vi "saveLogEntry.vi"(8 "error in (no error)":errorcluster, 11 "TestDataLog in":refnum<class "TestDataLog.lvclass">) -> (0 "error out":errorcluster, 3 "TestDataLog out":refnum<class "TestDataLog.lvclass">)   [LabVIEW 2016, in "TestDataLog.lvclass"]
uses:
  TestDataLog.lvclass
  D:/Code/ts_dcabt/Common_Log/Log/Log.lvclass
  TestDataLog.lvclass/TestDataLog.ctl
  Common_Log/Log/Log.lvclass/Log.ctl
  Common_Log/Log/Log.lvclass
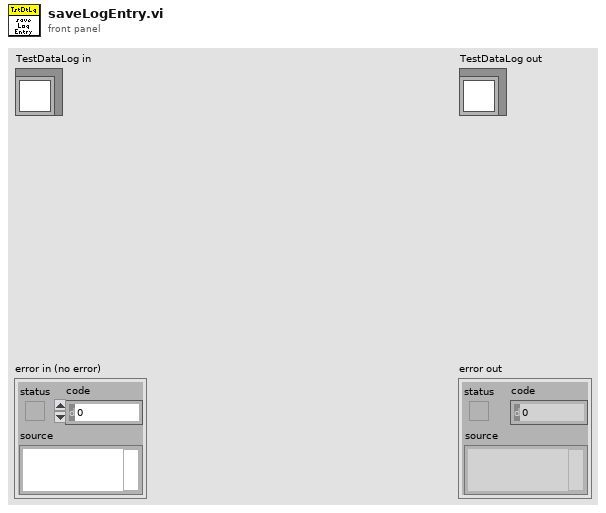
[diagram p1: front panel]
types:
  T1 = typedef "ILCBTTypedefs.lvlib/OutputData.ctl" = cluster{"Ch1":u16, "Ch2":u16, "Ch3":u16}
  T2 = typedef "ILCBTTypedefs.lvlib/StateSelector.ctl" = enum16{"EnabledState", "FaultState", "OffState", "StandbyState", "WaitingForTestState", "ExecutingTestState"}
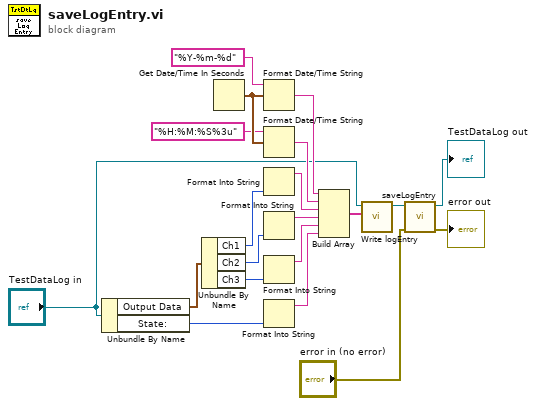
[diagram p0: block diagram]
diagram:
  n1 = Unbundle By Name("TestDataLog in") -> ("Output Data"=w20:T1, "State:"=w17:T2)
  n2 = Unbundle By Name(w20) -> ("Ch1"=w19:u16, "Ch2"=w5:u16, "Ch3"=w2:u16)
  n3 = Get Date/Time In Seconds() -> (seconds since 1Jan1904=w14:timestamp)
  n4 = Format Date/Time String(time format string (%c)="%Y-%m-%d" ("format string"), seconds (now)=w14) -> (date/time string=w11:string)  [unwired: 1 in]
  n5 = Format Date/Time String(time format string (%c)="%H:%M:%S%3u", seconds (now)=w14) -> (date/time string=w12:string)  [unwired: 1 in]
  n6 = Format Into String(w19) -> (resulting string=w18:string)  [unwired: 3 in, 1 out]
  n7 = Format Into String(w5) -> (resulting string=w4:string)  [unwired: 3 in, 1 out]
  n8 = Format Into String(w2) -> (resulting string=w3:string)  [unwired: 3 in, 1 out]
  n9 = Format Into String(w17) -> (resulting string=w16:string)  [unwired: 3 in, 1 out]
  n10 = Build Array(w11, w12, w18, w4, w3, w16) -> (w9:string[])
  n11 = call "Write logEntry.vi"("logEntry"=w9, "Logger in"="TestDataLog in") -> ("Logger out"=w10:refnum<class "TestDataLog.lvclass">)  [unwired: 9 in]
  n12 = call-parent "saveLogEntry.vi"("error in (no error)"="error in (no error)", "Logger in"=w10) -> ("error out"=→"error out":errorcluster, "Logger out"=→"TestDataLog out":refnum<class "TestDataLog.lvclass">)  [unwired: 8 in]
